vi "斐波纳契数列的递归算法(改进).vi"(9 "n":u32) -> (1 "F(n)":u32)   [LabVIEW 2021]
doc: "程序的说明请查看我的bl og： \nhttp://ruanqizhen.spaces.live.com/blog/cns!5852D4F797C53FB6!1832.entry"
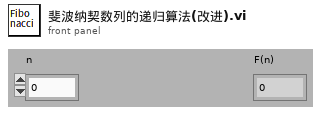
[diagram p1: front panel]
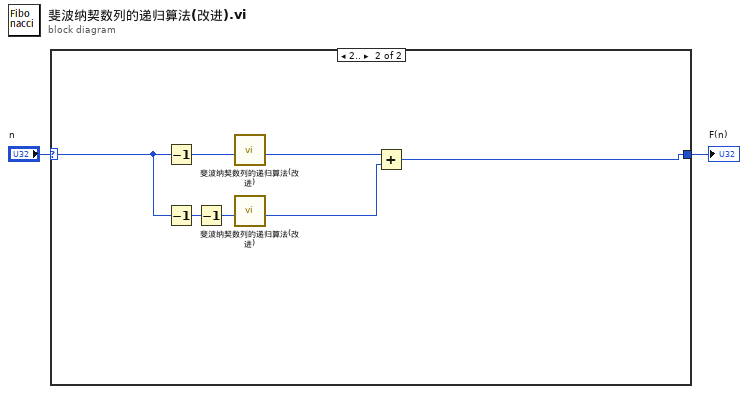
[diagram p0: block diagram]
diagram:
  n1 = case shown="2.." "n" {
    selector: "n" -> [w3 w10]
    tunnel: [w3 w8] -> w2
    frame ..1, Default {
    }
    frame 2.. {
      n2 = Decrement(x=w10) -> (x-1=w7:u32)
      n3 = Decrement(x=w10) -> (x-1=w9:u32)
      n4 = Decrement(x=w9) -> (x-1=w5:u32)
      n5 = call "斐波纳契数列的递归算法(改进).vi"("n"=w7) -> ("F(n)"=w6:u32)  [unwired: 10 in]
      n6 = call "斐波纳契数列的递归算法(改进).vi"("n"=w5) -> ("F(n)"=w4:u32)  [unwired: 10 in]
      n7 = Add(x=w6, y=w4) -> (x+y=w8:u32)
    }
  }
  "F(n)" <- w2
